vi "Get UI Details.vi"() -> ()   [LabVIEW 2021, in "Keysight 34461A DMM Measurement.lvlib"]
uses:
  Keysight 34461A DMM Measurement.lvlib
  <vilib>/Plug-In SDKs/Measurements/Helpers/TypeDefs/User Interface Information.ctl
  <vilib>/Plug-In SDKs/Measurements/NI Measurement Plug-In SDK.lvlib
  <vilib>/Utility/LVLibp/NI_PackedLibraryUtility.lvlib
panel:
  out "error out":errorcluster
  in  "error in (no error)":errorcluster
  out "user interface details":T1[](array[typedef])
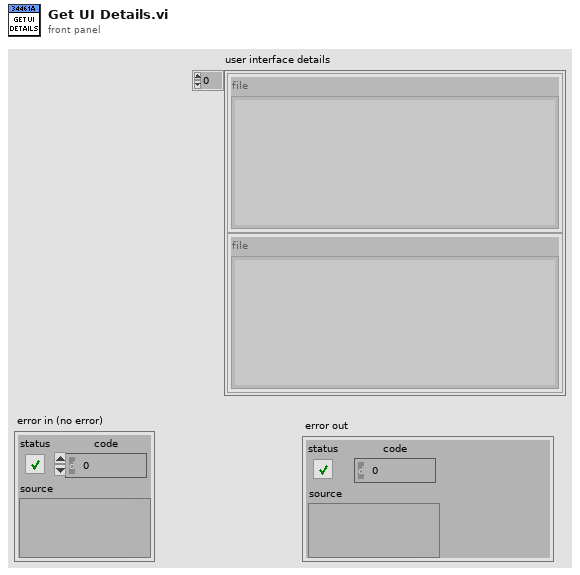
[diagram p1: front panel]
types:
  T1 = typedef "NI Measurement Plug-In SDK.lvlib/User Interface Information.ctl" = cluster{"file":string}
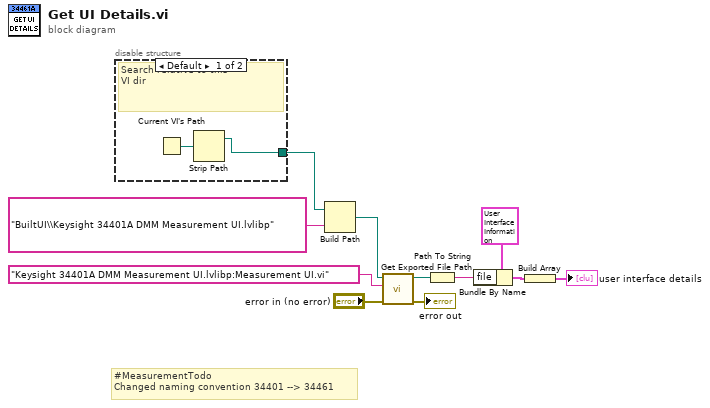
[diagram p0: block diagram]
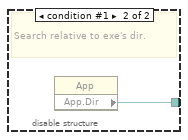
[diagram p2: hidden frame]
diagram:
  # "#MeasurementTodo\nChanged naming convention 34401 --> 34461"
  n1 = disable-structure shown="Default" {
    disable-tunnel: [w12 w14] -> w7
    frame condition #0 (active) {
      # "Search relative to this\nVI dir"
      n2 = Current VI's Path() -> (path=w13:path)
      n3 = Strip Path(path=w13) -> (stripped path=w12:path)  [unwired: 1 out]
    }
    frame condition #1 {
      # "Search relative to exe's dir."
      n4 = property class="App"() -> ("App.Dir"=w14:path)  [unwired: 2 in, 2 out]
    }
  }
  n5 = Build Path(base path=w7, name or relative path="BuiltUI\\Keysight 34401A DMM Measurement UI.lvlibp" ("file")) -> (appended path=w5:path)
  n6 = call <vilib>:"Get Exported File Path.vi"("error in (no error)"="error in (no error)", "qualified name"="Keysight 34401A DMM Measurement UI.lvlibp:Measurement UI.vi", "packed library path"=w5) -> ("error out"=→"error out":errorcluster, "path"=w2:path)  [unwired: 7 in]
  n7 = Path To String(path=w2) -> (string=w9:string)
  n8 = Bundle By Name(cluster=T1 {"file"="BuiltUI\\Keysight 34401A DMM Measurement UI.lvlibp\\Keysight 34401A DMM Measurement UI\\Measurement UI.vi"} ("UI Information"), "file"=w9) -> (w8:T1)
  n9 = Build Array(w8) -> (→"user interface details":T1[])
